vi "ABB Report Engineering Test.vi"(10 "Report in":string) -> (2 "Report out":string)   [LabVIEW 2017]
uses:
  <vilib>/Analysis/baseanly.llb/Mean (DBL).vi
  ABB global.vi
  <vilib>/Analysis/NI_AALBase.lvlib
panel:
  out "Ambient temp":dbl
  out "Efficiency Readings 2":dbl[][](array[numeric]) format="%#_4g"
  out "Efficiency Readings":dbl[][](array[numeric]) format="%#_4g"
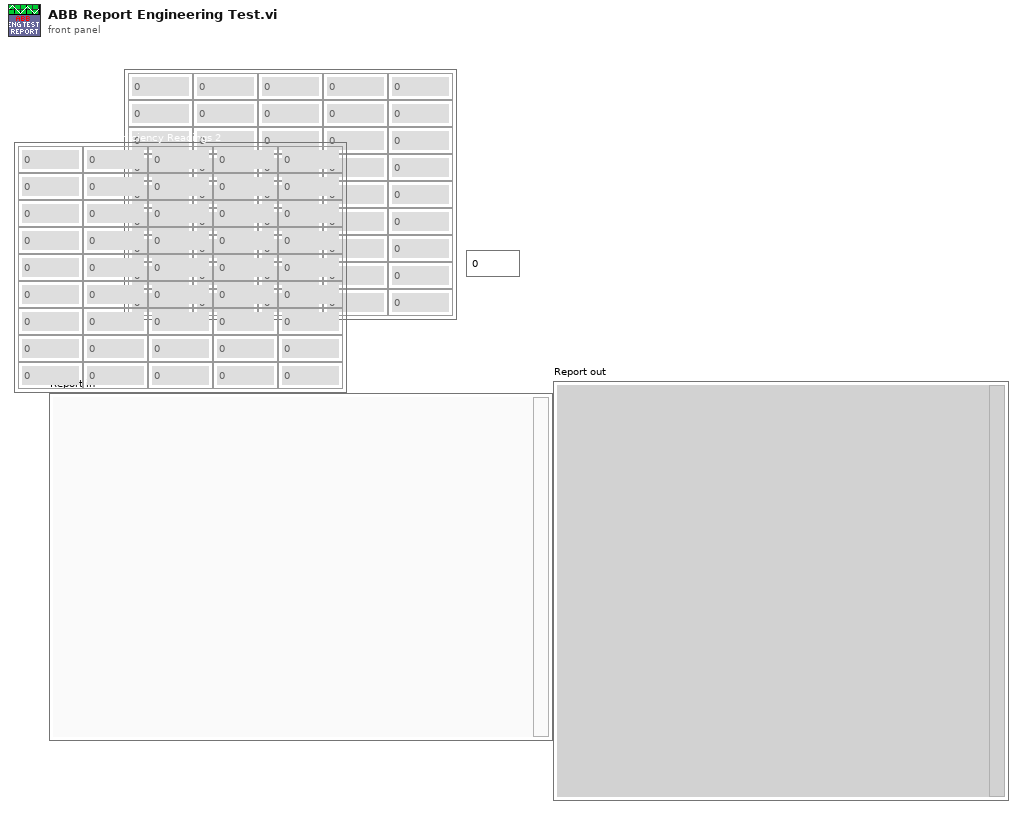
[diagram p1: front panel]
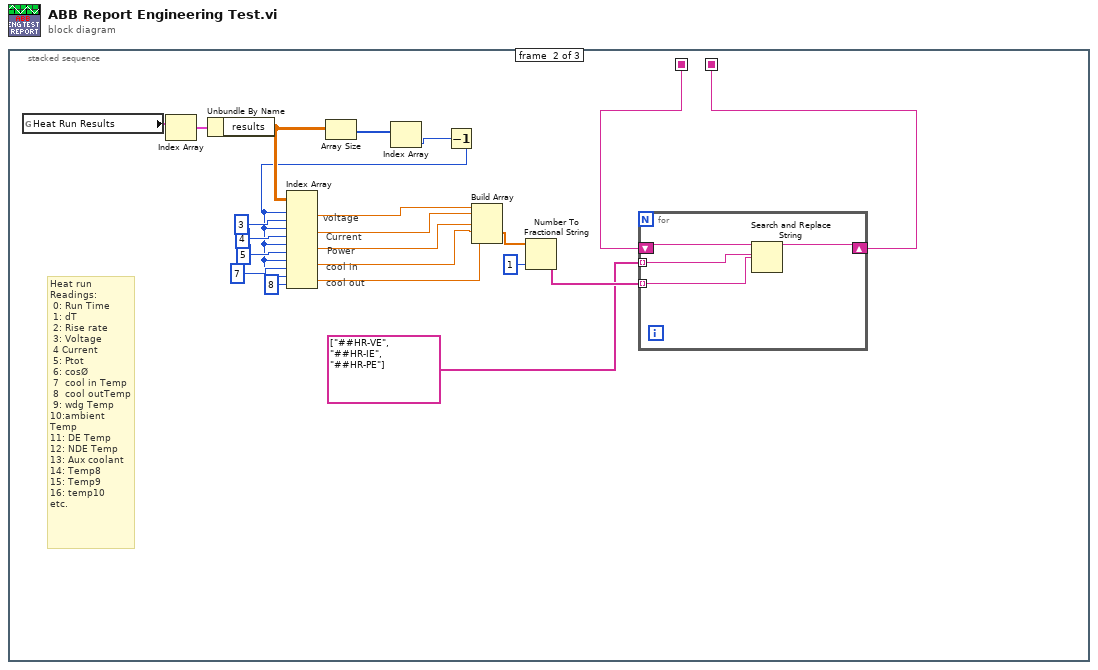
[diagram p0: block diagram]
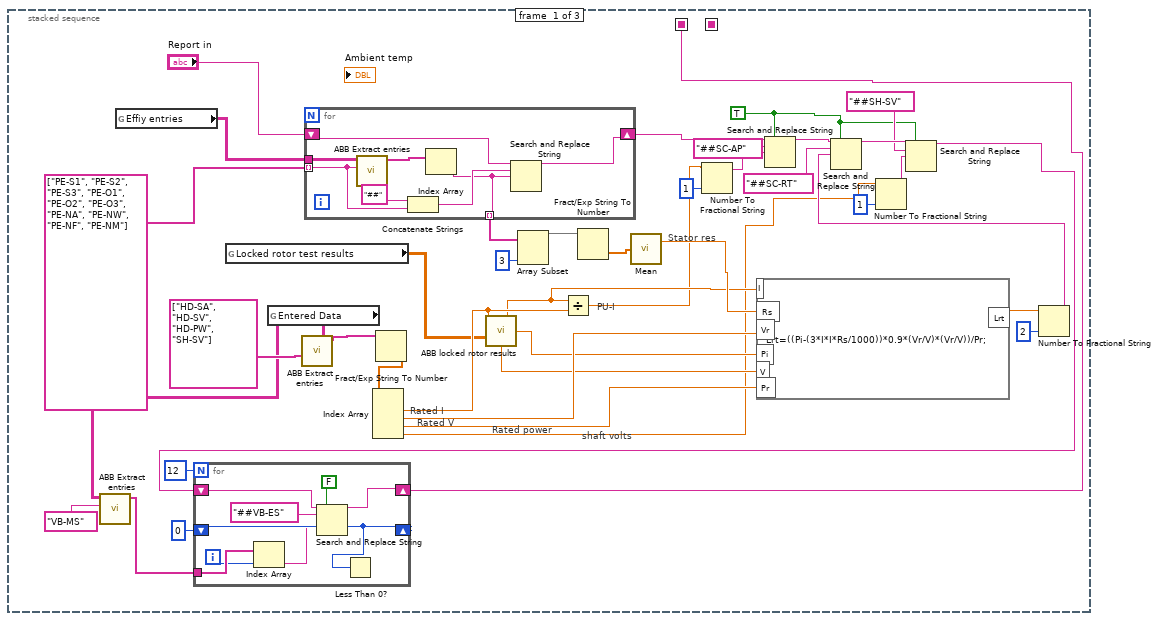
[diagram p2: hidden frame]
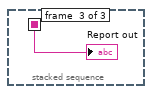
[diagram p3: hidden frame]
diagram:
  n1 = stacked-sequence {
    seq-local: [w9 _ _] -> [_ w64 _]
    seq-local: [_ w59 _] -> [_ _ w85]
    frame #0 {
      w4 = TRUE ("replace all? (F)")
      (unwired) string[] ["PE-S", "PE-M", "PE-I", "PE-C", "PE-R", "PE-Y", "PE-T", "PE-W", "PE-N"]
      (unwired) string[] ["PE-F", "PE-P", "PE-E"]
      # "shaft volts"
      # "Rated power"
      # "Rated V"
      # "Stator res"
      # "PU-I"
      # "Rated I"
      n2 = global read "ABB global.vi" "Effiy entries"() -> (w41:string[][])
      n3 = global read "ABB global.vi" "Locked rotor test results"() -> (w34:dbl[][])
      n4 = global read "ABB global.vi" "Entered Data"() -> (w10:string[][])
      n5 = call "ABB Extract entries.vi"("Entry ID"="VB-MS", "Entry table in"=w10) -> ("Selected Entries"=w13:string[])  [unwired: 9 in]
      n6 = call "ABB Extract entries.vi"("Entry IDs"=string[] ["HD-SA", "HD-SV", "HD-PW", "SH-SV"], "Entry table in"=w10) -> ("Selected Entries"=w37:string[])  [unwired: 9 in]
      n7 = for {
        tunnel: w41 -> [w58]
        tunnel: string[] ["PE-S1", "PE-S2", "PE-S3", "PE-O1", "PE-O2", "PE-O3", "PE-NA", "PE-NW", "PE-NF", "PE-NM"] -> [w54] mode=indexing
        shift-right: [w56] -> w14
        shift-left: "Report in" -> [w57]
        tunnel: [w51] -> w33 mode=indexing
        n8 = call "ABB Extract entries.vi"("Entry ID"=w54, "Entry table in"=w58) -> ("Selected Entries"=w55:string[])  [unwired: 9 in]
        n9 = Concatenate Strings("##", w54) -> (w52:string)
        n10 = Index Array(array=w55) -> (element=w51:string)  [unwired: 1 in]
        n11 = Search and Replace String(input string=w57, search string=w52, replace string=w51) -> (result string=w56:string)  [unwired: 5 in, 3 out]
      }
      n12 = Fract/Exp String To Number(string=w37) -> (number=w36:dbl[])  [unwired: 3 in, 1 out]
      n13 = Index Array(array=w36) -> (element #1=w35:dbl, element #2=w27:dbl, element #3=w24:dbl, element #4=w3:dbl)  [unwired: 4 in]
      n14 = call "ABB locked rotor results.vi"("Rated Current"=w35, "Locked rotor test results"=w34) -> ("I AVr"=w28:dbl, "PWr"=w26:dbl, "V AVr"=w25:dbl)  [unwired: 5 in, 6 out]
      n15 = Array Subset(array=w33, length=3) -> (w31:string[])  [unwired: 1 in]
      n16 = Divide(x=w28, y=w35) -> (x/y=w23:dbl)
      n17 = Fract/Exp String To Number(string=w31) -> (number=w30:dbl[])  [unwired: 3 in, 1 out]
      n18 = call-poly <vilib>:"Mean.vi"("X"=w30) -> ("mean"=w29:dbl)  [unwired: 1 out]
      n19 = Number To Fractional String(number=w23, precision (6)=i16 1) -> (F-format string=w21:string)  [unwired: 2 in]
      n20 = formula code="Lrt=((Pi-(3*I*I*Rs/1000))*0.9*(Vr/V)*(Vr/V))/Pr;"("I"=w28, "Rs"=w29, "Vr"=w27, "Pi"=w26, "V"=w25, "Pr"=w24) -> ("Lrt"=w18:dbl)
      n21 = Search and Replace String(replace all?=w4, input string=w14, search string="##SC-AP", replace string=w21) -> (result string=w19:string)  [unwired: 4 in, 3 out]
      n22 = Number To Fractional String(number=w3, precision (6)=i16 1) -> (F-format string=w1:string)  [unwired: 2 in]
      n23 = Number To Fractional String(number=w18, precision (6)=i16 2) -> (F-format string=w16:string)  [unwired: 2 in]
      n24 = Search and Replace String(replace all?=w4, input string=w19, search string="##SC-RT", replace string=w16) -> (result string=w7:string)  [unwired: 4 in, 3 out]
      n25 = Search and Replace String(replace all?=w4, input string=w7, search string="##SH-SV", replace string=w1) -> (result string=w6:string)  [unwired: 4 in, 3 out]
      n26 = for {
        N: 12 -> [_]
        shift-right: [w48] -> w9
        shift-left: w6 -> [w50]
        tunnel: w13 -> [w44]
        shift-right: [w45] -> _
        shift-left: 0 ("offset past replacement") -> [w47]
        i -> [w42]
        n27 = Index Array(array=w44, index=w42) -> (element=w43:string)
        n28 = Search and Replace String(replace all?=FALSE ("replace all? (F)"), input string=w50, search string="##VB-ES", replace string=w43, offset=w47) -> (result string=w48:string, offset past replacement=w45:i32)  [unwired: 3 in, 2 out]
        n29 = Less Than 0?(x=w45) -> ()  [unwired: 1 out]
      }
    }
    frame #1 {
      (unwired) string[] ["PE-S", "PE-M", "PE-I", "PE-C", "PE-R", "PE-Y", "PE-T", "PE-W", "PE-N"]
      (unwired) string[] ["PE-F", "PE-P", "PE-E"]
      # "cool out"
      # "cool in"
      # "Power"
      # "Current"
      # "voltage"
      # "Heat run Readings:\n 0: Run Time\n 1: dT\n 2: Rise rate\n 3: Voltage\n 4 Current\n 5: Ptot\n 6: cosØ\n 7  cool in Temp\n 8  cool outTemp\n 9: wdg Temp\n10:ambient Temp\n11: DE Temp\n12: NDE Temp\n13: Aux coolant\n14: Temp8\n15: Temp9\n16: temp10\netc."
      n30 = global read "ABB global.vi" "Heat Run Results"() -> (w80:cluster{"results":dbl[][], "Comments":string}[])
      n31 = Index Array(array=w80) -> (element=w79:cluster{"results":dbl[][], "Comments":string})  [unwired: 1 in]
      n32 = Unbundle By Name(w79) -> ("results"=w76:dbl[][])
      n33 = Array Size(array=w76) -> (size(s)=w78:i32[])
      n34 = Index Array(array=w78) -> (element=w77:i32)  [unwired: 1 in]
      n35 = Decrement(x=w77) -> (x-1=w71:i32)
      n36 = Index Array(array=w76, index (row) #1=w71, index (col) #1=3 ("disabled index (col)"), index (row) #2=w71, index (col) #2=4 ("disabled index (col)"), index (row) #3=w71, index (col) #3=5 ("disabled index (col)"), index (row) #4=w71, index (col) #4=7 ("disabled index (col)"), index (row) #5=w71, index (col) #5=8 ("disabled index (col)")) -> (element #1=w69:dbl, element #2=w68:dbl, element #3=w67:dbl, element #4=w66:dbl, element #5=w65:dbl)
      n37 = Build Array(w69, w68, w67, w66, w65) -> (w63:dbl[])
      n38 = Number To Fractional String(number=w63, precision (6)=i16 1) -> (F-format string=w61:string[])  [unwired: 2 in]
      n39 = for {
        shift-right: [w83] -> w59
        shift-left: w64 -> [w84]
        tunnel: w61 -> [w82] mode=indexing
        tunnel: string[] ["##HR-VE", "##HR-IE", "##HR-PE"] -> [w81] mode=indexing
        n40 = Search and Replace String(input string=w84, search string=w81, replace string=w82) -> (result string=w83:string)  [unwired: 5 in, 3 out]
      }
    }
    frame #2 {
      "Report out" <- w85
    }
  }
